vi "TEST_BinarySearch.vi"() -> ()   [LabVIEW 2024]
panel:
  out "Done":bool
  out "SP Guess":dbl
  in  "Unknown":dbl
  in  "Spec Lo":dbl
  in  "Spec HI":dbl
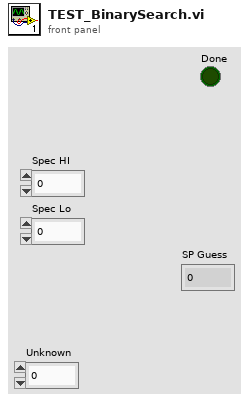
[diagram p1: front panel]
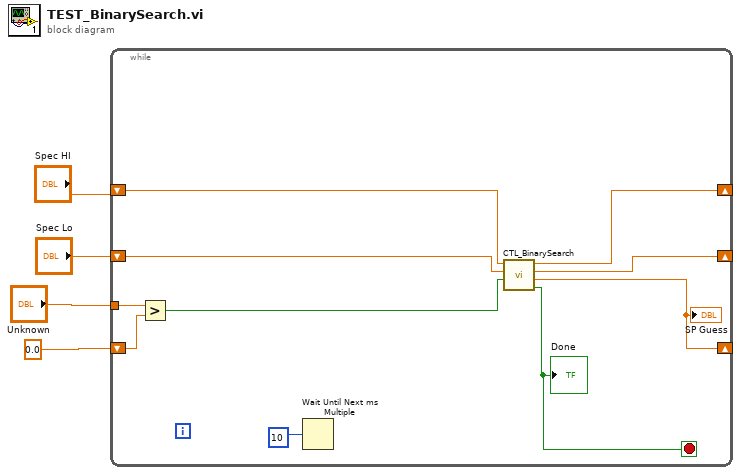
[diagram p0: block diagram]
diagram:
  n1 = while {
    shift-right: [w8] -> _
    shift-left: "Spec HI" -> [w11]
    shift-right: [w7] -> _
    shift-left: "Spec Lo" -> [w12]
    shift-right: [w6] -> _
    shift-left: 0.0 -> [w9]
    tunnel: "Unknown" -> [w10]
    stop <- w5 stop-if-true
    n2 = Greater?(x=w10, y=w9) -> (0:w13:bool)
    n3 = Wait Until Next ms Multiple(millisecond multiple=u32 10) -> ()  [unwired: 1 out]
    n4 = call "CTL_BinarySearch.vi"("Switched?"=w13, "Spec Lo in"=w12, "Spec HI in"=w11) -> ("Done"=w5:bool, "Guess"=w6:dbl, "Spec Lo out"=w7:dbl, "Spec HI out"=w8:dbl)  [unwired: 5 in]
    "SP Guess" <- w6
    "Done" <- w5
  }
